vi "COP Main.vi"() -> ()   [LabVIEW 2011]
uses:
  Support Files/VelocityState.ctl
  Support Files/TimeRec.ctl
  Support Files/LocalPose.ctl
  Support Files/Address.ctl
  Support Files/ServiceRec.ctl
  Support Files/RequestIDRec.ctl
  Support Files/ElementRec.ctl
  Support Files/LocalWaypointRec.ctl
  Support Files/JUDP Write Queue Element.ctl
  COP Support Files/COP FSM States.ctl
  <vilib>/Platform/TimedLoop/XDataNode/timing_clust.ctl
  <vilib>/Platform/TimedLoop/XDataNode/nitl_modes.ctl
  <vilib>/Platform/TimedLoop/XDataNode/wakeup.ctl
  cRIO/Functional Global Variables/Actions for FG's.ctl
  Support Files/JAUS Controller.ctl
  Support Files/Source ID Network Location Pair.ctl
  UDP Lib/UDP Network Location.ctl
  <vilib>/Platform/TimedLoop/XDataNode/XDataNode.xnode
  <vilib>/Platform/TimedLoop/XDataNode/XDNodeRunTimeDep.lvlib
panel:
  in  "Execute Waypoints":bool
  in  "Waypoints":T1
  out "Waypoint Request\nConfirmed":bool
  in  "Send Waypoints":bool
  in  "Logging?":bool=TRUE
  in  "RequestControl":bool
  in  "Resume":bool
  in  "Shutdown":bool
  in  "Standby":bool
  out "Robot's Controller":T4
  in  "Boolean":bool
  out "RBT Status":u8(ring) items=["INIT", "READY", "STANDBY", "SHUTDOWN", "FAILURE", "EMERGENCY"]
  out "Services":T5[](array[typedef])
  out "VI's Run States":T6(array[cluster])=[{"Name"="COP FSM.vi", "Exec.State"=enum."Idle"}, {"Name"="COP Logger.vi", "Exec.State"=enum."Idle"}]
  in  "Kill All":bool
  out "XY Graph":cluster{"Y":dbl[], "X":dbl[]}(graph)
  out "Robot ID":T4
  in  "COP ID":T4={"Subsystem Id"=124, "Node Id"=1, "Component Id"=1}
  out "LocalPose":T7
  out "VelocityState":T9
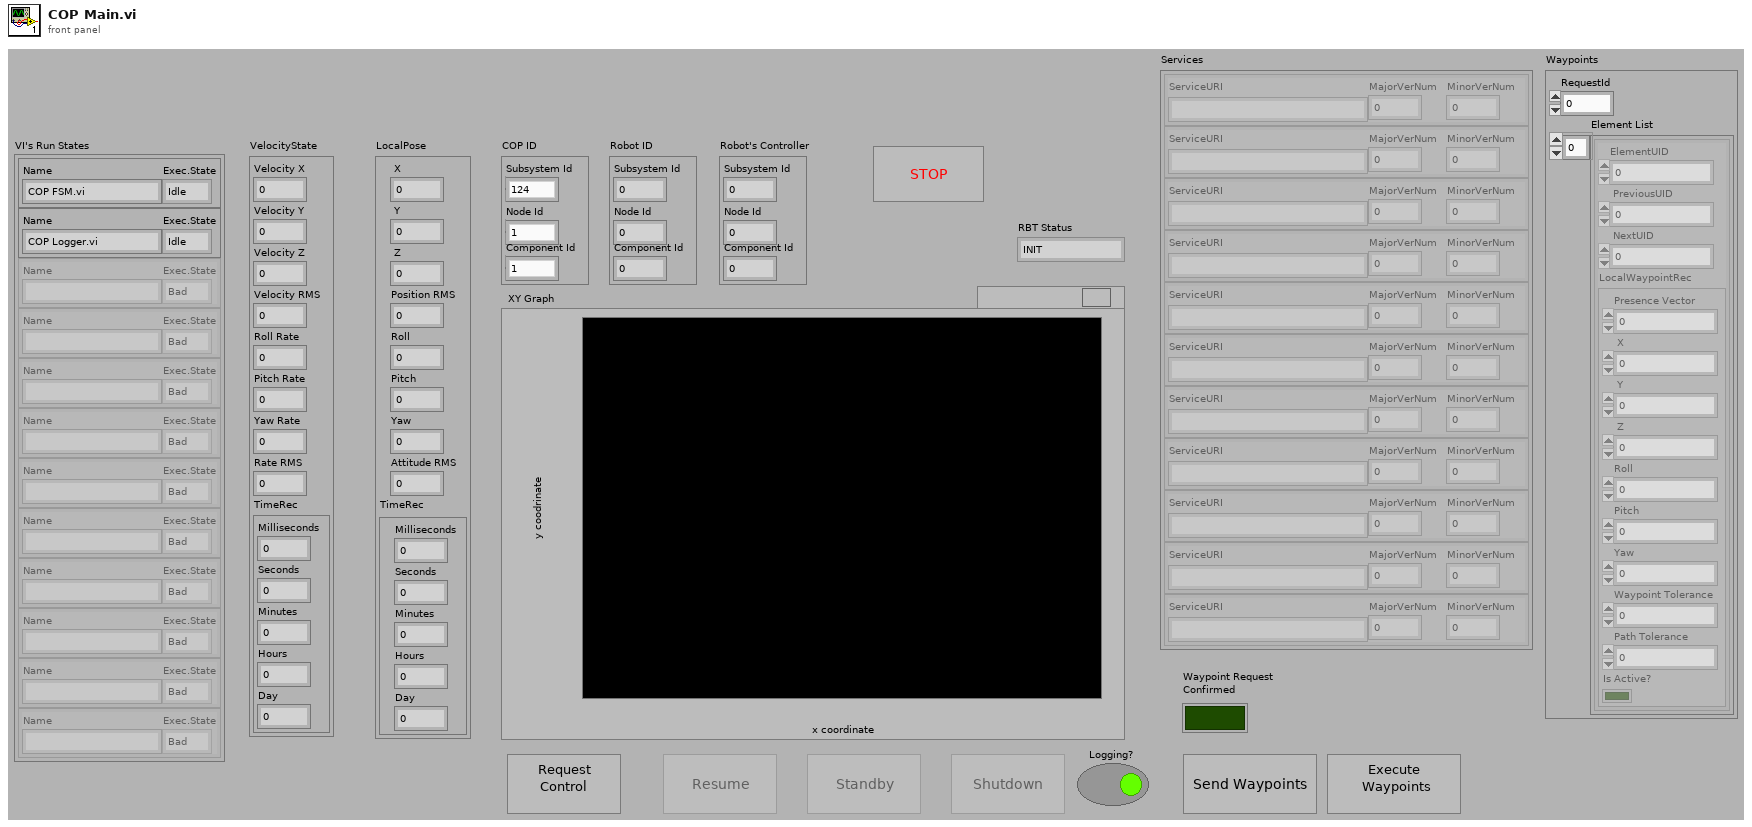
[diagram p1: front panel]
types:
  T1 = typedef "RequestIDRec.ctl" = cluster{"RequestId":u8, "Element List":T2[]}
  T2 = typedef "ElementRec.ctl" = cluster{"ElementUID":u16, " PreviousUID":u16, " NextUID":u16, "LocalWaypointRec":T3}
  T3 = typedef "LocalWaypointRec.ctl" = cluster{"Presence Vector":u8, " X":dbl, " Y":dbl, " Z":dbl, "Roll":dbl, "Pitch":dbl, "Yaw":dbl, "Waypoint Tolerance":dbl, "Path Tolerance":dbl, "Is Active?":bool}
  T4 = typedef "Address.ctl" = cluster{"Subsystem Id":u16, "Node Id":u8, "Component Id":u8}
  T5 = typedef "ServiceRec.ctl" = cluster{"ServiceURI":string, "MajorVerNum":u8, "MinorVerNum":u8}
  T6 = cluster{"Name":string, "Exec.State":enum32{"Bad", "Idle", "Run top level", "Running"}}[]
  T7 = typedef "LocalPose.ctl" = cluster{" X":dbl, " Y":dbl, " Z":dbl, "Position RMS":dbl, "Roll":dbl, "Pitch":dbl, "Yaw":dbl, "Attitude RMS":dbl, "TimeRec":T8}
  T8 = typedef "TimeRec.ctl" = cluster{"Milliseconds":u32, "Seconds":u32, "Minutes":u32, "Hours":u32, "Day":u32}
  T9 = typedef "VelocityState.ctl" = cluster{"Velocity X":dbl, "Velocity Y":dbl, "Velocity Z":dbl, "Velocity RMS":dbl, "Roll Rate":dbl, "Pitch Rate":dbl, "Yaw Rate":dbl, "Rate RMS":dbl, "TimeRec":T8}
  T10 = typedef "COP FSM States.ctl" = enum16{"QueryStatus", "rQueryIdentification", "sReportIdentification", "sQueryServices", "rReportServices", "sQueryControl", "rReportControl", "sRequestControl", "rConfirmControl", "sResume", "sStandby", "sShutdown", "sQueryVelocityState", "sQueryLocalPose", "rSendWaypoints", "rExecuteWaypoints"}
  T11 = typedef "JUDP Write Queue Element.ctl" = cluster{"Encoded JAUS Message":string, "Destination ID":u32}
  T12 = typedef "JAUS Controller.ctl" = cluster{"ID":T4, "Authority Code":u8}
  T13 = typedef "Source ID Network Location Pair.ctl" = cluster{"ID":u32, "Network Location":T14}
  T14 = typedef "UDP Network Location.ctl" = cluster{"IP Address":string, "Port":u16}
  T15 = typedef "Actions for FG's.ctl" = enum16{"Read", "Write"}
  T16 = typedef "XDNodeRunTimeDep.lvlib/timing_clust.ctl" = cluster{"Expected End [f-1]":u64, "Actual End [f-1]":u64, "Finished Late? [f-1]":bool, "Expected End [i-1]":u64, "Actual End [i-1]":u64, "Finished Late? [i-1]":bool, "Expected Start [i]":u64, "Actual Start [i]":u64, "Expected Start [f]":u64, "Actual Start [f]":u64, "Source Name":string, "Structure Name":string, "Period":i64, "Deadline":i64, "Offset":i64, "Start":i64, "Priority":i32, "Timeout":i32, "Mode":T17, "Wakeup Reason":T18, "Error":errorcluster, "Source Type":string, "Secondary Source Type":string, "Global End Time":u64, "Global Start Time":u64, "Frame Duration":u64, "Iteration Duration":u64, "Assigned CPU":i32, "I/O Scan Engine Mode":u32}
  T17 = typedef "XDNodeRunTimeDep.lvlib/nitl_modes.ctl" = enum32{"No Change", "Process missed periods, maintain original phase", "Discard missed periods, maintain original phase", "Process missed periods, ignore original phase", "Discard missed periods, ignore original phase"}
  T18 = typedef "XDNodeRunTimeDep.lvlib/wakeup.ctl" = enum32{"Normal", "Aborted", "Asynchronous wakeup", "Timing source error", "Timed loop error", "Timeout"}
  T19 = enum8{"Enabled", "Disabled", "Disabled and Grayed Out"}
  T20 = enum32{"Bad", "Idle", "Run top level", "Running"}
  T21 = cluster{"Name":string, "Exec.State":enum32{"Bad", "Idle", "Run top level", "Running"}}
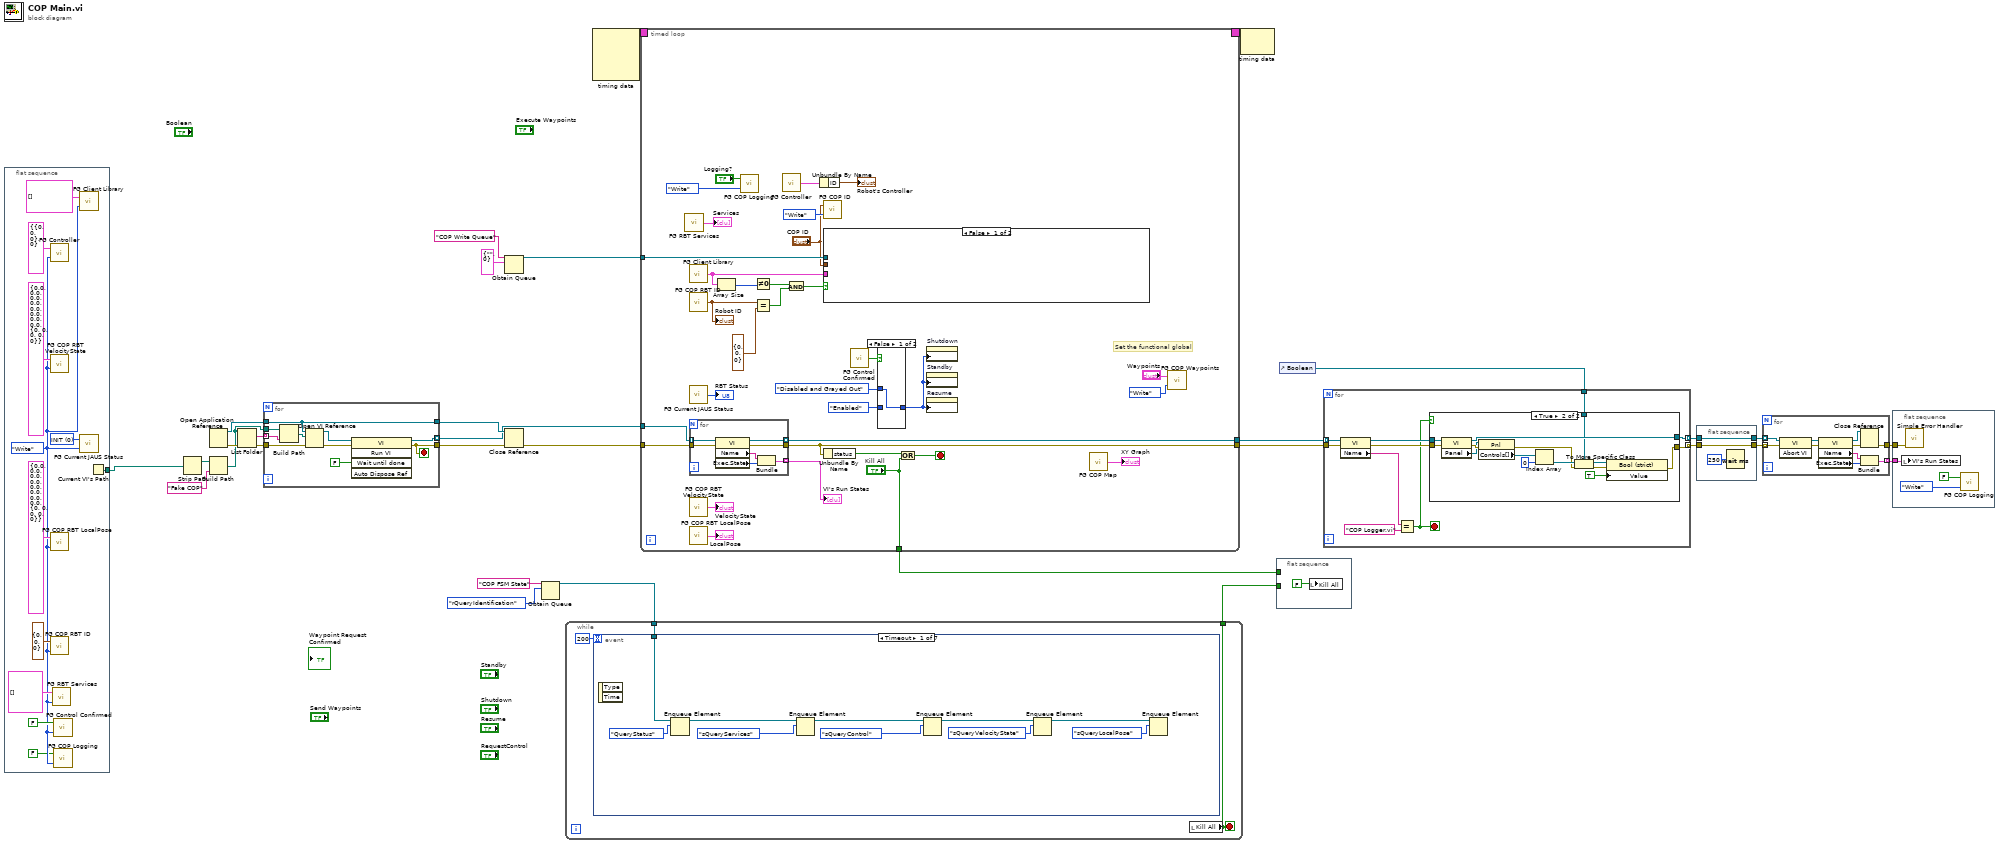
[diagram p0: block diagram]
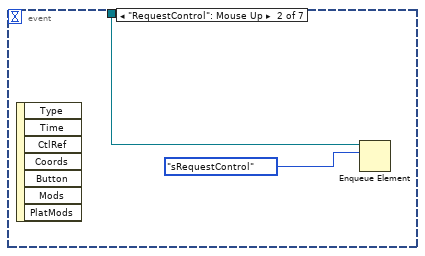
[diagram p2: hidden frame]
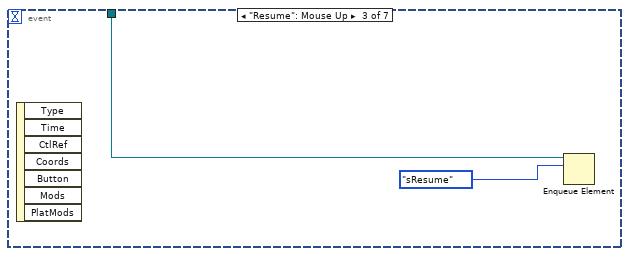
[diagram p3: hidden frame]
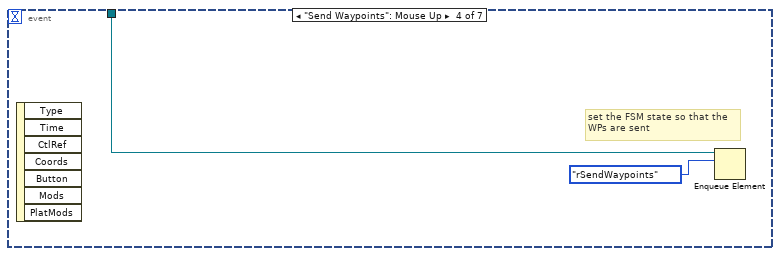
[diagram p4: hidden frame]
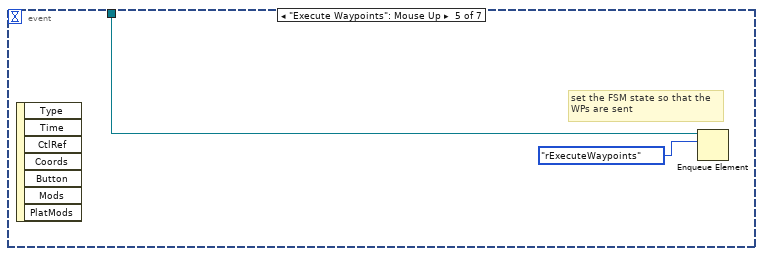
[diagram p5: hidden frame]
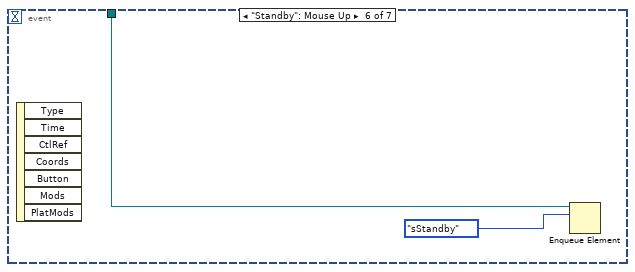
[diagram p6: hidden frame]
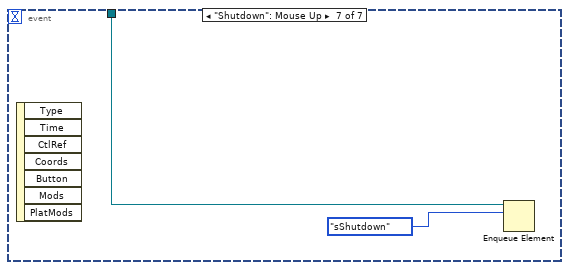
[diagram p7: hidden frame]
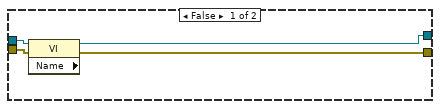
[diagram p8: hidden frame]
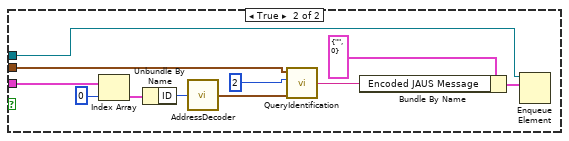
[diagram p10: hidden frame]
diagram:
  n1 = flat-sequence {
    tunnel: [w36] -> w1
    frame #0 {
      w33 = Actions_for_FG's."Write" ("FG Action (Read)")
      w40 = u8 0 items=["INIT", "READY", "STANDBY", "SHUTDOWN", "FAILURE", "EMERGENCY"] ("Status in")
      n2 = call "FG Controller.vi"("FG Action (Read)"=w33, "Controller in"=T12 {"ID"={"Subsystem Id"=0, "Node Id"=0, "Component Id"=0}, "Authority Code"=0}) -> ()  [unwired: 1 out]
      n3 = call "FG COP RBT VelocityState.vi"("FG Action (Read)"=w33, "RBT VelocityState in"=T9 {"Velocity X"=0.0, "Velocity Y"=0.0, "Velocity Z"=0.0, "Velocity RMS"=0.0, "Roll Rate"=0.0, "Pitch Rate"=0.0, "Yaw Rate"=0.0, "Rate RMS"=0.0, "TimeRec"={"Milliseconds"=0, "Seconds"=0, "Minutes"=0, "Hours"=0, "Day"=0}}) -> ()  [unwired: 1 out]
      n4 = call "FG COP RBT LocalPose.vi"("FG Action (Read)"=w33, "RBT LocalPose in"=T7 {" X"=0.0, " Y"=0.0, " Z"=0.0, "Position RMS"=0.0, "Roll"=0.0, "Pitch"=0.0, "Yaw"=0.0, "Attitude RMS"=0.0, "TimeRec"={"Milliseconds"=0, "Seconds"=0, "Minutes"=0, "Hours"=0, "Day"=0}}) -> ()  [unwired: 1 out]
      n5 = call "FG COP RBT ID.vi"("FG Action (Read)"=w33, "RBT ID in"=T4 {"Subsystem Id"=0, "Node Id"=0, "Component Id"=0}) -> ()  [unwired: 1 out]
      n6 = call "FG RBT Services.vi"("FG Action (Read)"=w33, "Services in"=T5[] []) -> ()  [unwired: 1 out]
      n7 = call "FG Control Confirmed.vi"("FG Action (Read)"=w33, "Control Confirmed in"=FALSE) -> ()  [unwired: 1 out]
      n8 = call "FG COP Logging.vi"("FG Action (Read)"=w33, "Logging? in"=FALSE) -> ()  [unwired: 1 out]
      n9 = call "FG Client Library.vi"("FG Action (Read)"=w33, "Client Records in"=T13[] []) -> ()  [unwired: 1 out]
      n10 = call "FG Current JAUS Status.vi"("FG Action (Read)"=w33, "Status in"=w40) -> ()  [unwired: 1 out]
      n11 = Current VI's Path() -> (path=w36:path)
    }
  }
  n12 = Strip Path(path=w1) -> (stripped path=w22:path)  [unwired: 1 out]
  n13 = Open Application Reference() -> (0:w27:errorcluster, 3:w29:refnum<vi>)  [unwired: 4 in]
  n14 = Build Path(base path=w22, name or relative path="Fake COP") -> (appended path=w21:path)
  n15 = List Folder(path=w21, error in=w27) -> (filenames=w28:string[], error out=w26:errorcluster)  [unwired: 2 in, 2 out]
  n16 = for {
    tunnel: w29 -> [w43]
    tunnel: w21 -> [w52]
    tunnel: w28 -> [w51] mode=indexing
    tunnel: w26 -> [w49]
    tunnel: [w47] -> w20 mode=indexing
    tunnel: [w44] -> w23
    tunnel: [w43] -> w24
    stop <- w44 stop-if-true
    n17 = Build Path(base path=w52, name or relative path=w51) -> (appended path=w50:path)
    n18 = Open VI Reference(application reference (local)=w43, vi path=w50, error in (no error)=w49) -> (vi reference=w48:refnum<vi>, error out=w46:errorcluster)  [unwired: 3 in]
    n19 = invoke class="VI" method="Run VI"(reference=w48, error in=w46, "Wait until done"=FALSE ("Wait Until Done")) -> (reference out=w47:refnum<vi>, error out=w44:errorcluster)  [unwired: 2 in, 3 out]
  }
  n20 = Obtain Queue(name (unnamed)="COP Write Queue", element data type=T11 {"Encoded JAUS Message"="", "Destination ID"=0} ("Cluster")) -> (queue out=w14:refnum<queue>)  [unwired: 3 in, 2 out]
  n21 = Close Reference(reference=w24, error in (no error)=w23) -> (error out=w19:errorcluster)
  n22 = Obtain Queue(name (unnamed)="COP FSM State", element data type=COP_FSM_States."rQueryIdentification" ("COP FSM States")) -> (queue out=w2:refnum<queue>)  [unwired: 3 in, 2 out]
  n23 = while {
    tunnel: [w54] -> w5
    tunnel: w2 -> [w53]
    stop <- w54 stop-if-true
    n24 = event shown="[0] Timeout" {
      selector: _ -> [_ _ _ _ _ _ _]
      dyn-events: _ -> [_ _ _ _ _ _ _]
      timeout: 200 -> [_ _ _ _ _ _ _]
      tunnel: w53 -> [w64 w67 w68 w71 w72 w74 w76]
      event Timeout {
        n25 = event-data() -> ()  [unwired: 1 in, 2 out]
        n26 = Enqueue Element(queue=w64, element=COP_FSM_States."QueryStatus") -> (queue out=w60:refnum<queue>)  [unwired: 2 in, 2 out]
        n27 = Enqueue Element(queue=w60, element=COP_FSM_States."sQueryServices") -> (queue out=w61:refnum<queue>)  [unwired: 2 in, 2 out]
        n28 = Enqueue Element(queue=w61, element=COP_FSM_States."sQueryControl") -> (queue out=w58:refnum<queue>)  [unwired: 2 in, 2 out]
        n29 = Enqueue Element(queue=w58, element=COP_FSM_States."sQueryVelocityState") -> (queue out=w57:refnum<queue>)  [unwired: 2 in, 2 out]
        n30 = Enqueue Element(queue=w57, element=COP_FSM_States."sQueryLocalPose") -> ()  [unwired: 2 in, 3 out]
      }
      event "RequestControl": Mouse Up {
        n31 = event-data() -> ()  [unwired: 1 in, 7 out]
        n32 = Enqueue Element(queue=w67, element=COP_FSM_States."sRequestControl") -> ()  [unwired: 2 in, 3 out]
      }
      event "Resume": Mouse Up {
        n33 = event-data() -> ()  [unwired: 1 in, 7 out]
        n34 = Enqueue Element(queue=w68, element=COP_FSM_States."sResume") -> ()  [unwired: 2 in, 3 out]
      }
      event "Send Waypoints": Mouse Up {
        # "set the FSM state so that the \nWPs are sent"
        n35 = event-data() -> ()  [unwired: 1 in, 7 out]
        n36 = Enqueue Element(queue=w71, element=COP_FSM_States."rSendWaypoints") -> ()  [unwired: 2 in, 3 out]
      }
      event "Execute Waypoints": Mouse Up {
        # "set the FSM state so that the \nWPs are sent"
        n37 = event-data() -> ()  [unwired: 1 in, 7 out]
        n38 = Enqueue Element(queue=w72, element=COP_FSM_States."rExecuteWaypoints") -> ()  [unwired: 2 in, 3 out]
      }
      event "Standby": Mouse Up {
        n39 = event-data() -> ()  [unwired: 1 in, 7 out]
        n40 = Enqueue Element(queue=w74, element=COP_FSM_States."sStandby") -> ()  [unwired: 2 in, 3 out]
      }
      event "Shutdown": Mouse Up {
        n41 = event-data() -> ()  [unwired: 1 in, 7 out]
        n42 = Enqueue Element(queue=w76, element=COP_FSM_States."sShutdown") -> ()  [unwired: 2 in, 3 out]
      }
    }
    n43 = local read "Kill All"() -> (w54:bool)
  }
  n44 = node-c288() -> (w31:T16)  [unwired: 4 in]
  n45 = timed-loop {
    tunnel: w20 -> [w108]
    tunnel: [w106] -> w13
    tunnel: w19 -> [w107]
    tunnel: [w105] -> w12
    timing: w31 -> [_]
    timing-out: [_] -> w30
    tunnel: w14 -> [w98]
    tunnel: ["Kill All"] -> w6
    stop <- w110 stop-if-true
    # "Set the functional global"
    n46 = call "FG RBT Services.vi"() -> ("Services out"=→"Services":T5[])  [unwired: 2 in]
    n47 = call "FG Client Library.vi"() -> ("Client Records out"=w92:T13[])  [unwired: 2 in]
    n48 = call "FG COP RBT ID.vi"() -> ("RBT ID out"=w93:T4)  [unwired: 2 in]
    "Robot ID" <- w93
    n49 = call "FG Current JAUS Status.vi"() -> ("Status out"=→"RBT Status":u8)  [unwired: 2 in]
    n50 = for {
      tunnel: w108 -> [w130] mode=indexing
      tunnel: w107 -> [w129]
      tunnel: [w126] -> w104 mode=indexing
      tunnel: [w125] -> w106 mode=indexing
      tunnel: [w124] -> w105
      n51 = property class="VI"(reference=w130, error in=w129) -> (reference out=w125:refnum<vi>, error out=w124:errorcluster, "Name"=w128:string, "Exec.State"=w127:T20)
      n52 = Bundle("Name"=w128, "Exec.State"=w127) -> (w126:T21)  [unwired: 1 in]
    }
    "VI's Run States" <- w104
    n53 = call "FG COP RBT VelocityState.vi"() -> ("RBT VelocityState out"=→"VelocityState":T9)  [unwired: 2 in]
    n54 = call "FG COP RBT LocalPose.vi"() -> ("RBT LocalPose out"=→"LocalPose":T7)  [unwired: 2 in]
    n55 = Array Size(array=w92) -> (size(s)=w96:i32)
    n56 = call "FG COP Logging.vi"("FG Action (Read)"=Actions_for_FG's."Write", "Logging? in"="Logging?") -> ()  [unwired: 1 out]
    n57 = Not Equal To 0?(x=w96) -> (x != 0?=w95:bool)
    n58 = Equal?(x=w93, y=T4 {"Subsystem Id"=0, "Node Id"=0, "Component Id"=0}) -> (x = y?=w99:bool)
    n59 = call "FG Controller.vi"() -> ("Controller out"=w89:T12)  [unwired: 2 in]
    n60 = And(x=w95, y=w99) -> (x .and. y?=w97:bool)
    n61 = Unbundle By Name(w89) -> ("ID"=→"Robot's Controller":T4)
    n62 = call "FG COP ID.vi"("FG Action (Read)"=Actions_for_FG's."Write", "COP ID in"="COP ID") -> ()  [unwired: 1 out]
    n63 = case shown="False" w97 {
      tunnel: w98 -> [_ w123]
      tunnel: "COP ID" -> [_ w118]
      tunnel: w92 -> [_ w117]
      frame False {
      }
      frame True {
        n64 = Index Array(array=w117, index=0) -> (element=w115:T13)
        n65 = Unbundle By Name(w115) -> ("ID"=w114:u32)
        n66 = call "AddressDecoder.vi"("Address"=w114) -> ("Address Cluster"=w113:T4)
        n67 = call "QueryIdentification.vi"("Destination"=w113, "QueryType"=u8 2, "Source"=w118) -> ("Encoded JAUS Message"=w120:string)  [unwired: 1 in]
        n68 = Bundle By Name(cluster=T11 {"Encoded JAUS Message"="", "Destination ID"=0} ("Cluster"), "Encoded JAUS Message"=w120) -> (w121:T11)
        n69 = Enqueue Element(queue=w123, element=w121) -> ()  [unwired: 2 in, 3 out]
      }
    }
    n70 = Unbundle By Name(w105) -> ("status"=w109:bool)
    n71 = call "FG Control Confirmed.vi"() -> ("Control Confirmed out"=w86:bool)  [unwired: 2 in]
    n72 = case shown="False" w86 {
      tunnel: T19."Enabled" ("Disabled") -> [_ w112]
      tunnel: T19."Disabled and Grayed Out" ("Disabled") -> [w111 _]
      tunnel: [w111 w112] -> w83
      frame False {
      }
      frame True {
      }
    }
    n73 = Or(x=w109, y="Kill All") -> (x .or. y?=w110:bool)
    n74 = property on="Shutdown" class="Bool (strict)"("DisabledEnum"=w83) -> ()  [unwired: 2 in, 2 out]
    n75 = property on="Standby" class="Bool (strict)"("DisabledEnum"=w83) -> ()  [unwired: 2 in, 2 out]
    n76 = property on="Resume" class="Bool (strict)"("DisabledEnum"=w83) -> ()  [unwired: 2 in, 2 out]
    n77 = call "FG COP Map.vi"() -> ("Map out"=→"XY Graph":cluster{"Y":dbl[], "X":dbl[]})  [unwired: 2 in]
    n78 = call "FG COP Waypoints.vi"("FG Action (Read)"=Actions_for_FG's."Write", "COP Waypoints in"="Waypoints") -> ()  [unwired: 1 out]
  }
  n79 = node-c288(w30) -> ()  [unwired: 1 out]
  n80 = flat-sequence {
    tunnel: w6 -> [_]
    tunnel: w5 -> [_]
    frame #0 {
      n81 = local write "Kill All"(FALSE ("Kill All")) -> ()
    }
  }
  n82 = control-ref of="Boolean"() -> (w11:refnum<vi>)
  n83 = for {
    tunnel: w13 -> [w143] mode=indexing
    tunnel: w12 -> [w140]
    tunnel: [w137] -> w9 mode=indexing
    tunnel: [w136] -> w8 mode=indexing
    tunnel: w11 -> [w135]
    stop <- w134 stop-if-true
    n84 = property class="VI"(reference=w143, error in=w140) -> (reference out=w139:refnum<vi>, error out=w138:errorcluster, "Name"=w142:string)
    n85 = Equal?(x=w142, y="COP Logger.vi") -> (x = y?=w134:bool)
    n86 = case shown="True" w134 {
      tunnel: w139 -> [w147 w161]
      tunnel: w138 -> [w146 w160]
      tunnel: [w145 w148] -> w137
      tunnel: [w144 w157] -> w136
      tunnel: w135 -> [_ w152]
      frame False {
        n87 = property class="VI" props=["Name"](reference=w147, error in=w146) -> (reference out=w144:refnum<vi>, error out=w145:errorcluster)  [unwired: 1 out]
      }
      frame True {
        n88 = property class="VI"(reference=w161, error in=w160) -> (reference out=w157:refnum<vi>, error out=w159:errorcluster, "Panel"=w158:refnum<vi>)
        n89 = property class="Pnl"(reference=w158, error in=w159) -> (error out=w149:errorcluster, "Controls[]"=w156:refnum<vi>[])  [unwired: 1 out]
        n90 = Index Array(array=w156, index=0) -> (element=w154:refnum<vi>)
        n91 = To More Specific Class(target class=w152, reference=w154, error in=w149) -> (specific class reference=w153:refnum<vi>, error out=w150:errorcluster)
        n92 = property on="Property Node" class="Bool (strict)"(reference=w153, error in=w150, "Value"=TRUE) -> (error out=w148:errorcluster)  [unwired: 1 out]
      }
    }
  }
  n93 = flat-sequence {
    tunnel: [w163] -> w10
    tunnel: w9 -> [w163]
    tunnel: w8 -> [w162]
    tunnel: [w162] -> w7
    frame #0 {
      n94 = Wait (ms)(milliseconds to wait=u32 250) -> ()  [unwired: 1 out]
    }
  }
  n95 = for {
    tunnel: w7 -> [w174] mode=indexing
    tunnel: w10 -> [w173] mode=indexing
    tunnel: [w166] -> w18 mode=indexing
    tunnel: [w165] -> w17
    n96 = invoke class="VI" method="Abort VI"(reference=w174, error in=w173) -> (reference out=w170:refnum<vi>, error out=w169:errorcluster)  [unwired: 1 in, 1 out]
    n97 = property class="VI"(reference=w170, error in=w169) -> (reference out=w168:refnum<vi>, error out=w167:errorcluster, "Name"=w171:string, "Exec.State"=w172:T20)
    n98 = Close Reference(reference=w168, error in (no error)=w167) -> (error out=w165:errorcluster)
    n99 = Bundle("Name"=w171, "Exec.State"=w172) -> (w166:T21)  [unwired: 1 in]
  }
  n100 = flat-sequence {
    tunnel: w18 -> [w178]
    tunnel: w17 -> [w177]
    frame #0 {
      n101 = local write "VI's Run States"(w178) -> ()
      n102 = call <vilib>:"Simple Error Handler.vi"("error in (no error)"=w177) -> ()  [unwired: 4 in, 5 out]
      n103 = call "FG COP Logging.vi"("FG Action (Read)"=Actions_for_FG's."Write", "Logging? in"=FALSE) -> ()  [unwired: 1 out]
    }
  }
